vi "Array_Size_1D.vi"(10 "Array":i8[](array[numeric])=[0, 1, 2, 3]) -> (2 "Size":i32)   [LabVIEW 2018]
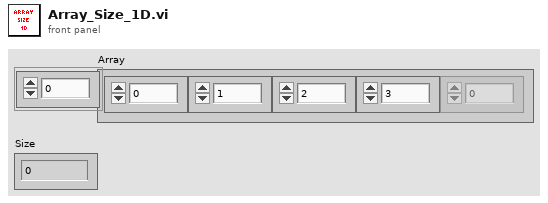
[diagram p1: front panel]
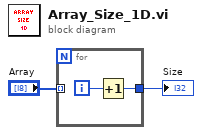
[diagram p0: block diagram]
diagram:
  n1 = for {
    tunnel: "Array" -> [_] mode=indexing
    tunnel: [w3] -> w2
    i -> [w4]
    n2 = Increment(x=w4) -> (x+1=w3:i32)
  }
  "Size" <- w2
